vi "Operation Window.vi"(6 "Main UI Message Queue":refnum<queue>, 7 "Pump On?":enum16{"Off", "On", "Not Initialized"}(ring), 8 "error in (no error)":errorcluster, 9 "Graph Notifier":refnum<notifier>, 10 "Message Queues":T24, 11 "Feed Module State Cluster in":T2={"Shared Variables"={"PID 1 Process Variable"="PID1-Mettler Toledo Scale 1", "PID 1 Output"="PID1-Mettler Toledo Scale 1", "PID 1 Setpoint"="PID1-Setpoint", "PID 1 Setpoint SV refnum"="ni.var.psp://localhost/Flow Module 1/PID1-Setpoint", "PID 1 Process Variable SV refnum"="ni.var.psp://localhost/Flow Module 1/PID1-Setpoint", "PID 1 Output SV refnum"="ni.var.psp://localhost/Flow Module 1/PID1-Setpoint"}, "Feed Module Config"={"GUID"="", "Drop Coords"={"Horizontal"=0, "Vertical"=0}, "Process Name"="", "Queue Name"="", "Settings"={"Cycle Period"=500.0, "Ismatech"={"VISA resource name"="", "Simulated?"=TRUE, "Pump Number"=1.0, "Reverse?"=FALSE}, "Masterflex"={"VISA resource name"="", "Simulated?"=TRUE, "Pump Number"=1.0, "Reverse?"=FALSE}, "Mettler"={"VISA resource name"="", "Simulated?"=FALSE}, "Bronkhorst M13 Flow Meter"={"VISA resource name"="", "Simulated?"=TRUE, "Smoothing Steps"=1}, "PID 2 Parameters"={"Input Device"=enum."Default", "Output Device"=enum."Default", "Setpoint"=0.0, "PID gains"={"proportional gain (Kc)"=1.0, "integral time (Ti, min)"=0.01, "derivative time (Td, min)"=0.0}}, "Manual Entry"=0.0, "Auto?"=TRUE, "output range"={"output high"=100.0, "output low"=0.0}, "Tacmina Settings"={"Analog DAQ Task"="", "Digital DAQ Task"=""}, "KNF SIMDOS Settings"={"VISA resource name"="", "Simulated?"=TRUE}, "ASIA Pump C"={"ASIA Pump #"=0, "channel"=0, "Simulated"=FALSE}, "VICI Settings"={"VISA resource name"="", "Simulated?"=TRUE, "Pump Letter"="", "Reverse?"=FALSE}, "FLOM Settings"={"VISA resource name"="", "Simulated?"=TRUE, "Pump Number"=0.0}, "SSI PR/LD Settings"={"VISA resource name"="", "Simulated?"=FALSE}, "Masterflex 75211 Settings"={"Analog DAQ Task"="", "Digital DAQ Task"=""}, "SSI P40 Settings"={"VISA resource name"="", "Simulated?"=TRUE}, "Ismatech 3 Channel Settings"={"VISA resource name"="", "Pump Number"=1, "Channel Number"=0, "Simulated?"=TRUE, "Reverse?"=FALSE}, "Bronkhorst M14 Settings"={"VISA resource name"="", "Simulated?"=FALSE, "Smoothing Steps"=1}}, "Settings Load Count"=0, "OP Load Count"=0}} {"Feed Module Config"."Settings"."Bronkhorst M14 Settings"."Smoothing Steps" min=1 step=1; "Feed Module Config"."Settings"."Ismatech 3 Channel Settings"."Channel Number" min=0 max=3; "Feed Module Config"."Settings"."Ismatech 3 Channel Settings"."Pump Number" min=1; "Feed Module Config"."Settings"."output range"."output low" min=0.0 max=100.0 format="%.2f"; "Feed Module Config"."Settings"."output range"."output high" format="%.2f"; "Feed Module Config"."Settings"."PID 2 Parameters"."PID gains"."derivative time (Td, min)" format="%.3f"; "Feed Module Config"."Settings"."PID 2 Parameters"."PID gains"."integral time (Ti, min)" format="%.3f"; "Feed Module Config"."Settings"."PID 2 Parameters"."PID gains"."proportional gain (Kc)" format="%.3f"; "Feed Module Config"."Settings"."Bronkhorst M13 Flow Meter"."Smoothing Steps" min=1 step=1; "Feed Module Config"."Settings"."ASIA Pump C"."channel" min=0 max=1 step=1; "Feed Module Config"."Settings"."Ismatech"."Pump Number" min=1.0 max=20.0 step=1.0; "Feed Module Config"."Settings"."Masterflex"."Pump Number" min=1.0 max=20.0 step=1.0}) -> (0 "error out":errorcluster, 2 "Need Update":bool, 3 "Feed Module State Cluster out":T2={"Shared Variables"={"PID 1 Process Variable"="PID1-Mettler Toledo Scale 1", "PID 1 Output"="PID1-Mettler Toledo Scale 1", "PID 1 Setpoint"="PID1-Setpoint", "PID 1 Setpoint SV refnum"="ni.var.psp://localhost/Flow Module 1/PID1-Setpoint", "PID 1 Process Variable SV refnum"="ni.var.psp://localhost/Flow Module 1/PID1-Setpoint", "PID 1 Output SV refnum"="ni.var.psp://localhost/Flow Module 1/PID1-Setpoint"}, "Feed Module Config"={"GUID"="", "Drop Coords"={"Horizontal"=0, "Vertical"=0}, "Process Name"="", "Queue Name"="", "Settings"={"Cycle Period"=500.0, "Ismatech"={"VISA resource name"="", "Simulated?"=TRUE, "Pump Number"=1.0, "Reverse?"=FALSE}, "Masterflex"={"VISA resource name"="", "Simulated?"=TRUE, "Pump Number"=1.0, "Reverse?"=FALSE}, "Mettler"={"VISA resource name"="", "Simulated?"=FALSE}, "Bronkhorst M13 Flow Meter"={"VISA resource name"="", "Simulated?"=TRUE, "Smoothing Steps"=1}, "PID 2 Parameters"={"Input Device"=enum."Default", "Output Device"=enum."Default", "Setpoint"=0.0, "PID gains"={"proportional gain (Kc)"=1.0, "integral time (Ti, min)"=0.01, "derivative time (Td, min)"=0.0}}, "Manual Entry"=0.0, "Auto?"=TRUE, "output range"={"output high"=100.0, "output low"=0.0}, "Tacmina Settings"={"Analog DAQ Task"="", "Digital DAQ Task"=""}, "KNF SIMDOS Settings"={"VISA resource name"="", "Simulated?"=TRUE}, "ASIA Pump C"={"ASIA Pump #"=0, "channel"=0, "Simulated"=FALSE}, "VICI Settings"={"VISA resource name"="", "Simulated?"=TRUE, "Pump Letter"="", "Reverse?"=FALSE}, "FLOM Settings"={"VISA resource name"="", "Simulated?"=TRUE, "Pump Number"=0.0}, "SSI PR/LD Settings"={"VISA resource name"="", "Simulated?"=FALSE}, "Masterflex 75211 Settings"={"Analog DAQ Task"="", "Digital DAQ Task"=""}, "SSI P40 Settings"={"VISA resource name"="", "Simulated?"=TRUE}, "Ismatech 3 Channel Settings"={"VISA resource name"="", "Pump Number"=1, "Channel Number"=0, "Simulated?"=TRUE, "Reverse?"=FALSE}, "Bronkhorst M14 Settings"={"VISA resource name"="", "Simulated?"=FALSE, "Smoothing Steps"=1}}, "Settings Load Count"=0, "OP Load Count"=0}} {"Feed Module Config"."Settings"."Bronkhorst M14 Settings"."Smoothing Steps" min=1 step=1; "Feed Module Config"."Settings"."Ismatech 3 Channel Settings"."Channel Number" min=0 max=3; "Feed Module Config"."Settings"."Ismatech 3 Channel Settings"."Pump Number" min=1; "Feed Module Config"."Settings"."output range"."output low" min=0.0 max=100.0 format="%.2f"; "Feed Module Config"."Settings"."output range"."output high" format="%.2f"; "Feed Module Config"."Settings"."PID 2 Parameters"."PID gains"."derivative time (Td, min)" format="%.3f"; "Feed Module Config"."Settings"."PID 2 Parameters"."PID gains"."integral time (Ti, min)" format="%.3f"; "Feed Module Config"."Settings"."PID 2 Parameters"."PID gains"."proportional gain (Kc)" format="%.3f"; "Feed Module Config"."Settings"."Bronkhorst M13 Flow Meter"."Smoothing Steps" min=1 step=1; "Feed Module Config"."Settings"."ASIA Pump C"."channel" min=0 max=1 step=1; "Feed Module Config"."Settings"."Ismatech"."Pump Number" min=1.0 max=20.0 step=1.0; "Feed Module Config"."Settings"."Masterflex"."Pump Number" min=1.0 max=20.0 step=1.0})   [LabVIEW 2018, in "Feed Module.lvlib"]
uses:
  Feed Module/Feed Module.lvlib
  Feed Module/Controls/Feed Message Queues.ctl
  support/Message Queue/Message Cluster.ctl
  Feed Module/Controls/Feed Module State Cluster.ctl
  Feed Module/Controls/Feed Module Shared Variable Cluster.ctl
  Feed Module/Controls/Feed Module Config Cluster.ctl
  <vilib>/Utility/miscctls.llb/LVPoint32TypeDef.ctl
  Feed Module/Controls/Feed Module Settings Cluster.ctl
  Ismatec ISM 831C/Controls/Ismatech ISM831C Settings Cluster.ctl
  Masterflex 7550-30/Controls/Settings Cluster.ctl
  Mettler Toledo/Controls/Settings Cluster.ctl
  Bronkhorst M13 Flow Meter/Settings Cluster.ctl
  Measure Instrument/PID 2 Parameters Cluster.ctl
  Measure Instrument/PID Input Enum.ctl
  Measure Instrument/PID 2 Output Enum.ctl
  Tacmina QI/Tacmina QI DAQ Setting.ctl
  KNF Pump/Settings Cluster plus SIMDOS.ctl
  ASIA Pump/Pump Settings.ctl
  VICI M50 Party Mode/Settings Cluster.ctl
  FLOM Pump/Settings Cluster.ctl
  SSI PR Class/SSI PR or LD Settings Cluster.ctl
  Masterflex 75211/Masterflex 75211 DAQ Setting.ctl
  SSI PR Class/SSI P40 Settings Cluster.ctl
  Ismatec 78001/Ismatec 4083.ctl
  Bronkhorst M14 Flow Meter/Settings Cluster.ctl
  Config Module/Controls/OP Window Display.ctl
  support/Message Queue/Enqueue Message (Single).vi
  support/Message Queue/Message Queue.lvlib
  support/Support Library.lvlib
  Settings/Settings Dialog.vi
  Settings/Settings.lvlib
  Ismatec ISM 831C/Ismatec ISM 831C.lvlib
  Masterflex 7550-30/Masterflex 7550-30.lvlib
  Mettler Toledo/Mettler Toledo.lvlib
  Bronkhorst M13 Flow Meter/Bronkhorst M13 Flow Meter.lvlib
  Tacmina QI/Tacmina QI.lvlib
  KNF Pump/KNF SIMDOS.lvlib
  ASIA Pump.lvlib
  VICI M50 Party Mode/VICI M6 M50 Party Mode.lvlib
  FLOM Pump/FLOM Pump.lvlib
  SSI PR Class/SSI PR or LD Pump.lvlib
  Masterflex 75211/Masterflex 75211.lvlib
  SSI PR Class/SSI P40 Pump.lvlib
  Ismatec 78001/Ismatec 4308.lvlib
  Bronkhorst M14 Flow Meter/Bronkhorst M14 Flow Meter.lvlib
panel:
  out "Smoothed Array":dbl[](array[numeric])
  out "Start button status":T1(ring)
  out "Started":bool
  out "Updated":bool
  out "Flow":dbl caption="gm/min" format="%.2f"
  out "Data":waveform(dbl)[](graph)
  in  "Auto?":bool=TRUE
  in  "Manual Entry":dbl step=0.1 format="%#_6f"
  in  "Setpoint":dbl
  in  "Cancel Button":bool
  in  "OK Button":bool
  in  "Start":bool
  in  "Settings":bool
  in  "Stop":bool
  # "Output Instruments"
  # "Input Instruments"
  # "Output Instruments"
  # "Input Instruments"
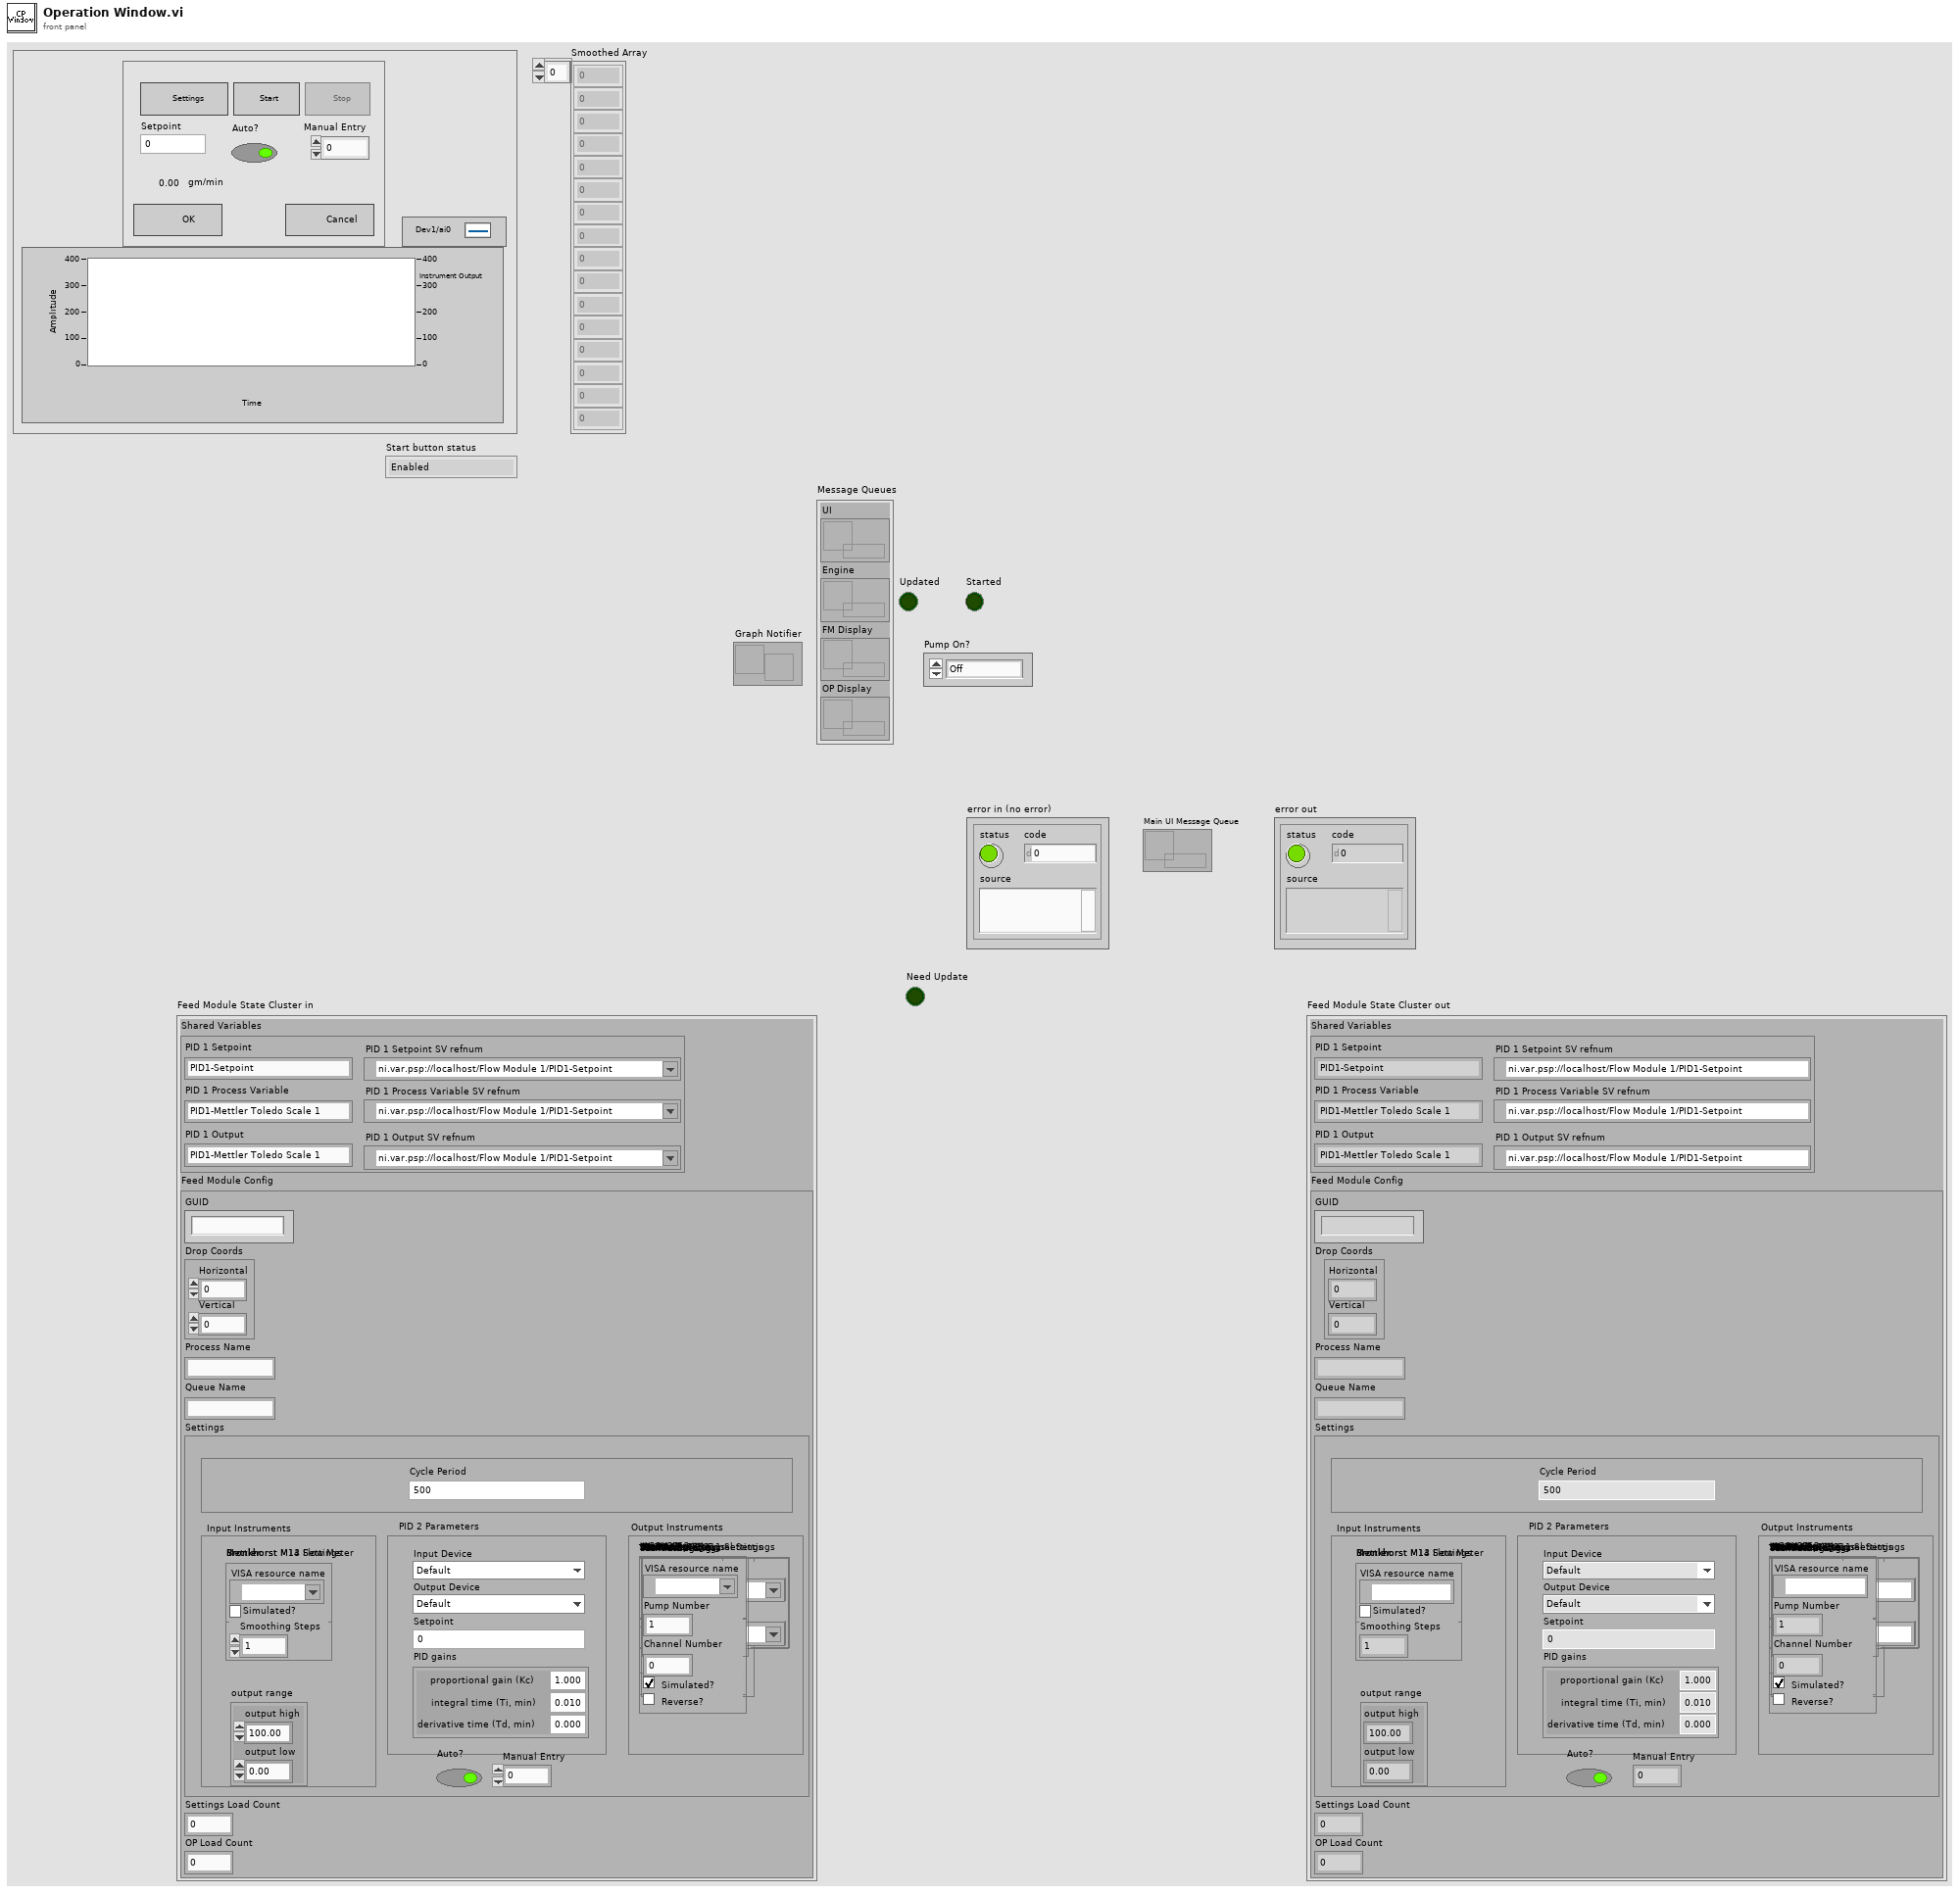
[diagram p1: front panel]
types:
  T1 = enum8{"Enabled", "Disabled", "Disabled and Grayed Out"}
  T2 = typedef "Feed Module.lvlib/Feed Module State Cluster.ctl" = cluster{"Shared Variables":T3, "Feed Module Config":T4}
  T3 = typedef "Feed Module.lvlib/Feed Module Shared Variable Cluster.ctl" = cluster{"PID 1 Process Variable":string, "PID 1 Output":string, "PID 1 Setpoint":string, "PID 1 Setpoint SV refnum":refnum<k21>, "PID 1 Process Variable SV refnum":refnum<k21>, "PID 1 Output SV refnum":refnum<k21>}
  T4 = typedef "Feed Module.lvlib/Feed Module Config Cluster.ctl" = cluster{"GUID":string, "Drop Coords":T5, "Process Name":string, "Queue Name":string, "Settings":T6, "Settings Load Count":i32, "OP Load Count":i32}
  T5 = typedef "LVPoint32TypeDef.ctl" = cluster{"Horizontal":i32, "Vertical":i32}
  T6 = typedef "Feed Module.lvlib/Feed Module Settings Cluster.ctl" = cluster{"Cycle Period":dbl, "Ismatech":T7, "Masterflex":T8, "Mettler":T9, "Bronkhorst M13 Flow Meter":T10, "PID 2 Parameters":T11, "Manual Entry":dbl, "Auto?":bool, "output range":cluster{"output high":dbl, "output low":dbl}, "Tacmina Settings":T14, "KNF SIMDOS Settings":T15, "ASIA Pump C":T16, "VICI Settings":T17, "FLOM Settings":T18, "SSI PR/LD Settings":T19, "Masterflex 75211 Settings":T20, "SSI P40 Settings":T21, "Ismatech 3 Channel Settings":T22, "Bronkhorst M14 Settings":T23}
  T7 = typedef "Ismatec ISM 831C.lvlib/Ismatech ISM831C Settings Cluster.ctl" = cluster{"VISA resource name":refnum<visa-resource-name>, "Simulated?":bool, "Pump Number":dbl, "Reverse?":bool}
  T8 = typedef "Masterflex 7550-30.lvlib/Settings Cluster.ctl" = cluster{"VISA resource name":refnum<visa-resource-name>, "Simulated?":bool, "Pump Number":dbl, "Reverse?":bool}
  T9 = typedef "Mettler Toledo.lvlib/Settings Cluster.ctl" = cluster{"VISA resource name":refnum<visa-resource-name>, "Simulated?":bool}
  T10 = typedef "Bronkhorst M13 Flow Meter.lvlib/Settings Cluster.ctl" = cluster{"VISA resource name":refnum<visa-resource-name>, "Simulated?":bool, "Smoothing Steps":i32}
  T11 = typedef "PID 2 Parameters Cluster.ctl" = cluster{"Input Device":T12, "Output Device":T13, "Setpoint":dbl, "PID gains":cluster{"proportional gain (Kc)":dbl, "integral time (Ti, min)":dbl, "derivative time (Td, min)":dbl}}
  T12 = typedef "PID Input Enum.ctl" = enum16{"Default", "Bronkhorst M13", "Bronkhorst M14", "Scale Rate of Change"}
  T13 = typedef "PID 2 Output Enum.ctl" = enum16{"Default", "Ismatec ISM 4308", "Ismatec ISM 831C", "Masterflex 7550-30", "VICI", "Tacmina QI", "KNF SIMDOS", "ASIA Type C", "FLOM UI-22-11", "SSI PR/LD", "SSI P40", "Masterflex 75211-70"}
  T14 = typedef "Tacmina QI.lvlib/Tacmina QI DAQ Setting.ctl" = cluster{"Analog DAQ Task":refnum<k21>, "Digital DAQ Task":refnum<k21>}
  T15 = typedef "KNF SIMDOS.lvlib/Settings Cluster plus SIMDOS.ctl" = cluster{"VISA resource name":refnum<visa-resource-name>, "Simulated?":bool}
  T16 = typedef "ASIA Pump.lvlib/Pump Settings.ctl" = cluster{"ASIA Pump #":i32, "channel":i32, "Simulated":bool}
  T17 = typedef "VICI M6 M50 Party Mode.lvlib/Settings Cluster.ctl" = cluster{"VISA resource name":refnum<visa-resource-name>, "Simulated?":bool, "Pump Letter":string, "Reverse?":bool}
  T18 = typedef "FLOM Pump.lvlib/Settings Cluster.ctl" = cluster{"VISA resource name":refnum<visa-resource-name>, "Simulated?":bool, "Pump Number":dbl}
  T19 = typedef "SSI PR or LD Pump.lvlib/SSI PR or LD Settings Cluster.ctl" = cluster{"VISA resource name":refnum<visa-resource-name>, "Simulated?":bool}
  T20 = typedef "Masterflex 75211.lvlib/Masterflex 75211 DAQ Setting.ctl" = cluster{"Analog DAQ Task":refnum<k21>, "Digital DAQ Task":refnum<k21>}
  T21 = typedef "SSI P40 Pump.lvlib/SSI P40 Settings Cluster.ctl" = cluster{"VISA resource name":refnum<visa-resource-name>, "Simulated?":bool}
  T22 = typedef "Ismatec 4308.lvlib/Ismatec 4083.ctl" = cluster{"VISA resource name":refnum<visa-resource-name>, "Pump Number":i16, "Channel Number":i16, "Simulated?":bool, "Reverse?":bool}
  T23 = typedef "Bronkhorst M14 Flow Meter.lvlib/Settings Cluster.ctl" = cluster{"VISA resource name":refnum<visa-resource-name>, "Simulated?":bool, "Smoothing Steps":i32}
  T24 = typedef "Feed Module.lvlib/Feed Message Queues.ctl" = cluster{"UI":refnum<queue>, "Engine":refnum<queue>, "FM Display":refnum<queue>, "OP Display":refnum<queue>}
  T25 = typedef "Feed Module.lvlib/OP Window Display.ctl" = cluster{"Flow":dbl, "Manual":dbl, "Pump Status":u16, "Smoothed Array":dbl[]}
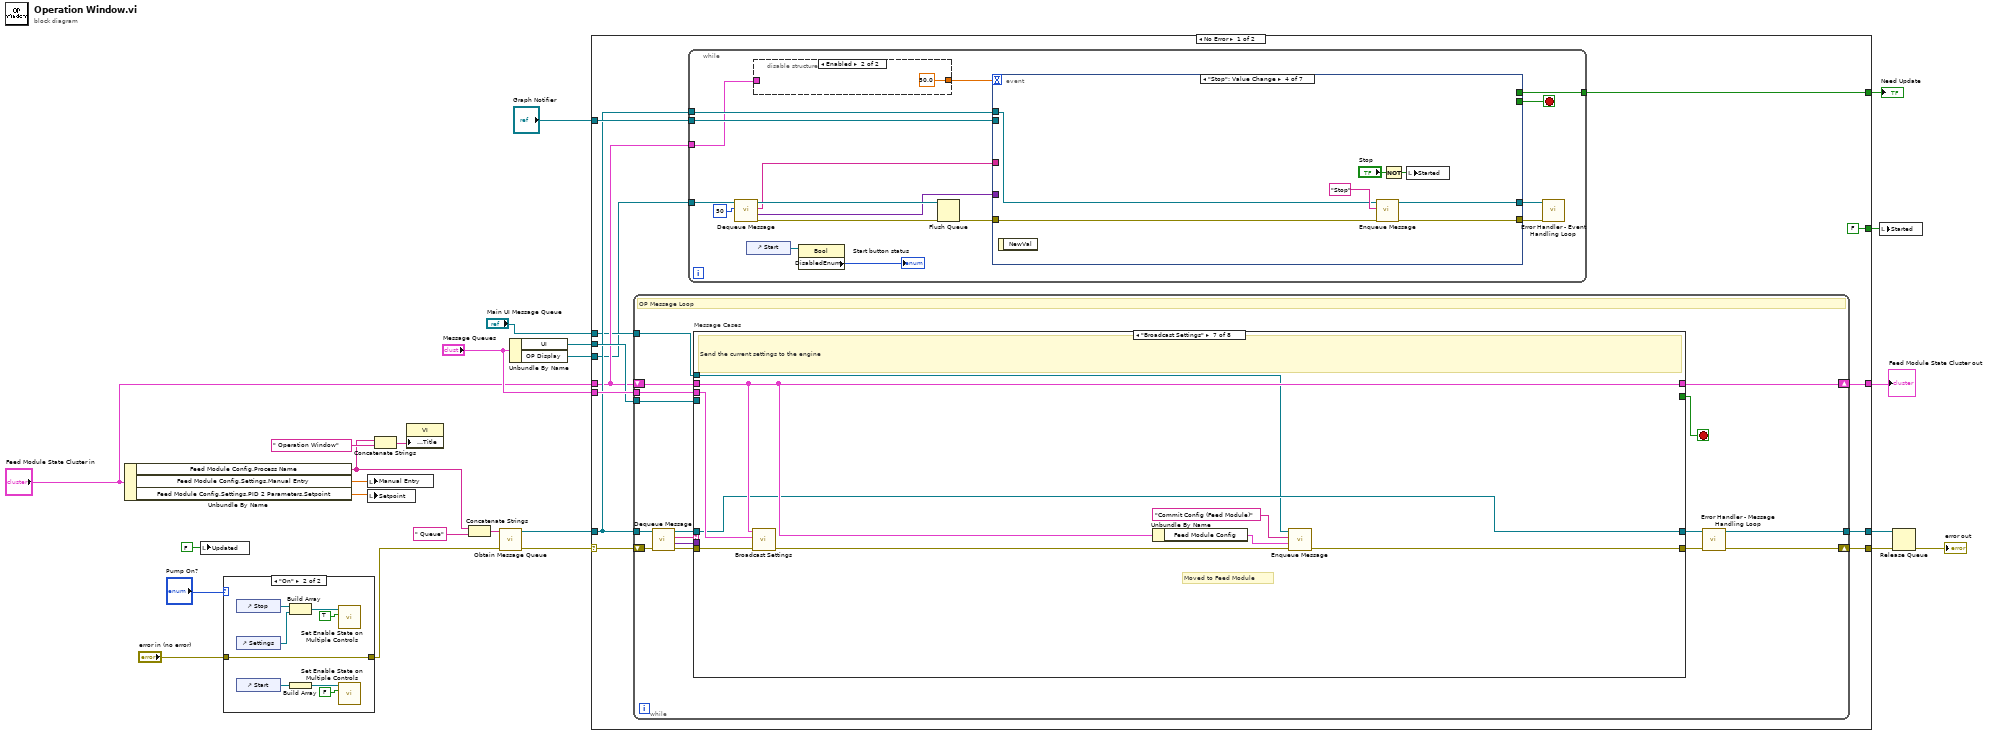
[diagram p0: block diagram]
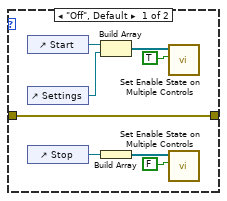
[diagram p2: hidden frame]
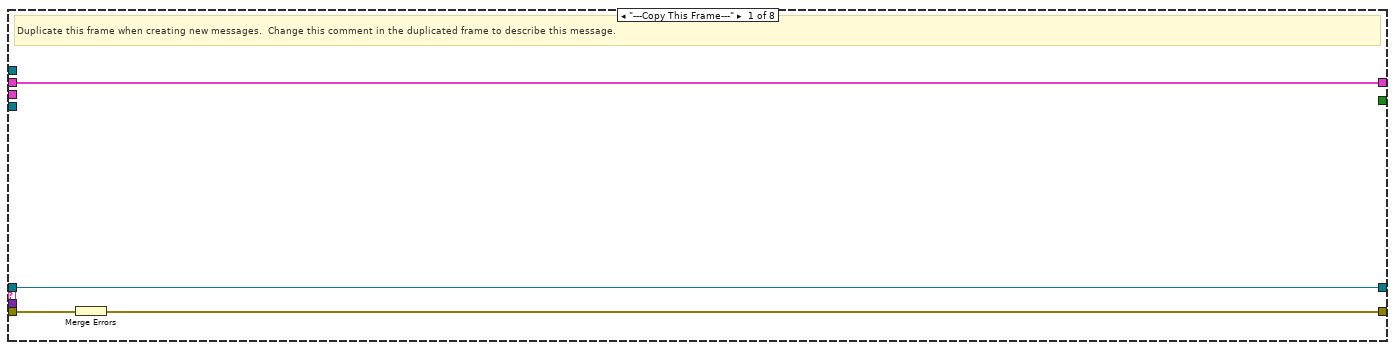
[diagram p3: hidden frame]
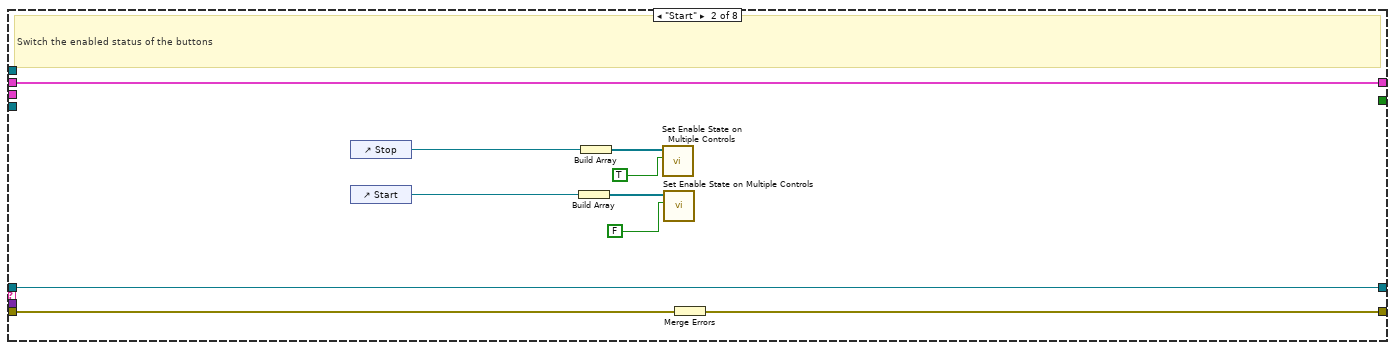
[diagram p4: hidden frame]
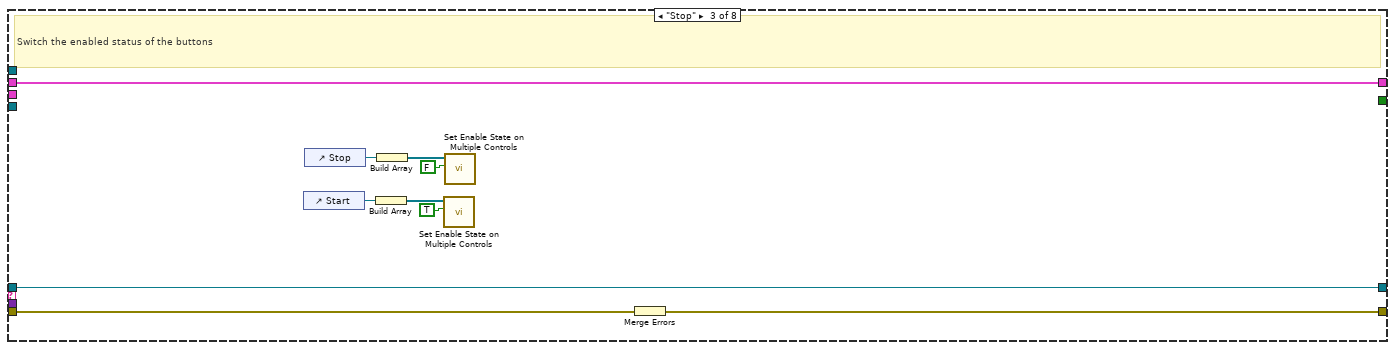
[diagram p5: hidden frame]
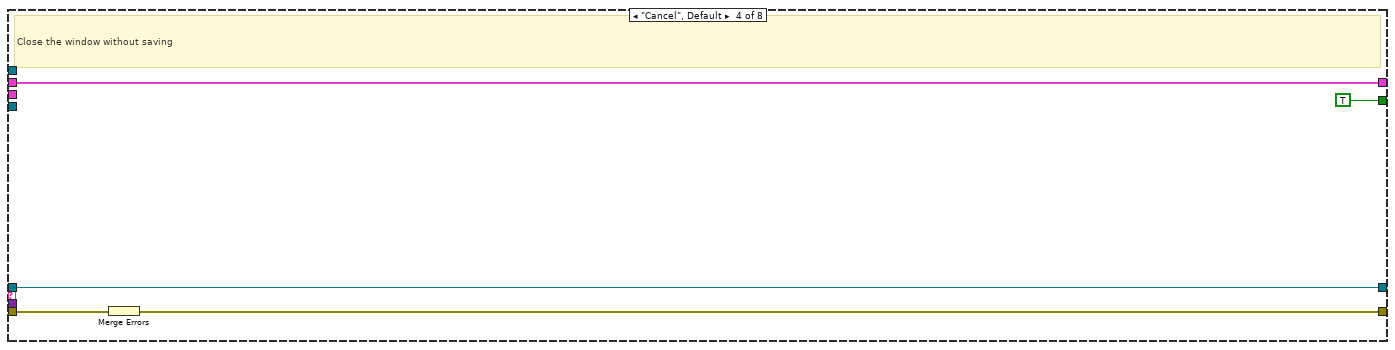
[diagram p6: hidden frame]
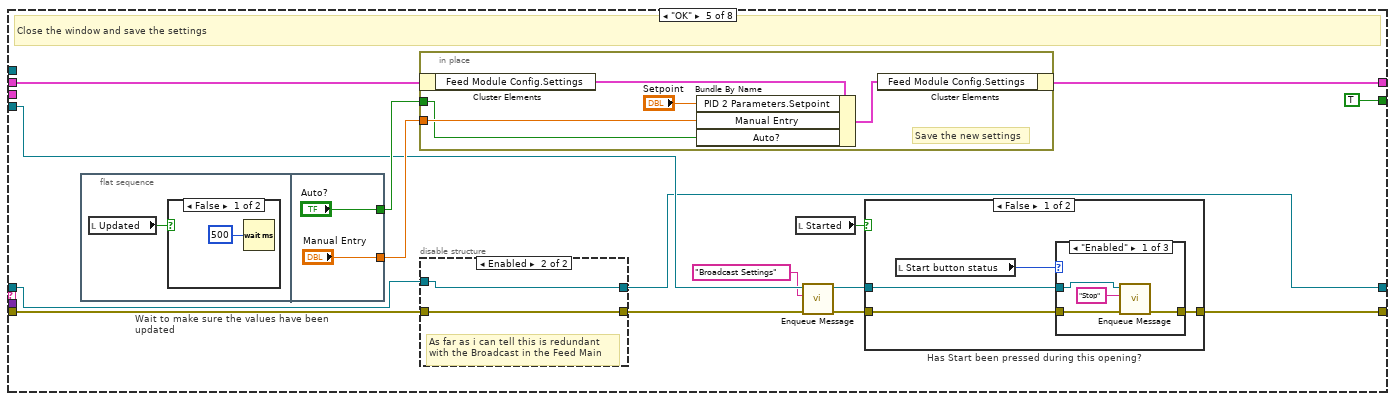
[diagram p7: hidden frame]
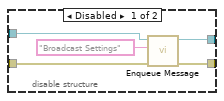
[diagram p8: hidden frame]
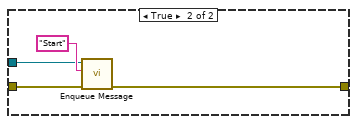
[diagram p11: hidden frame]
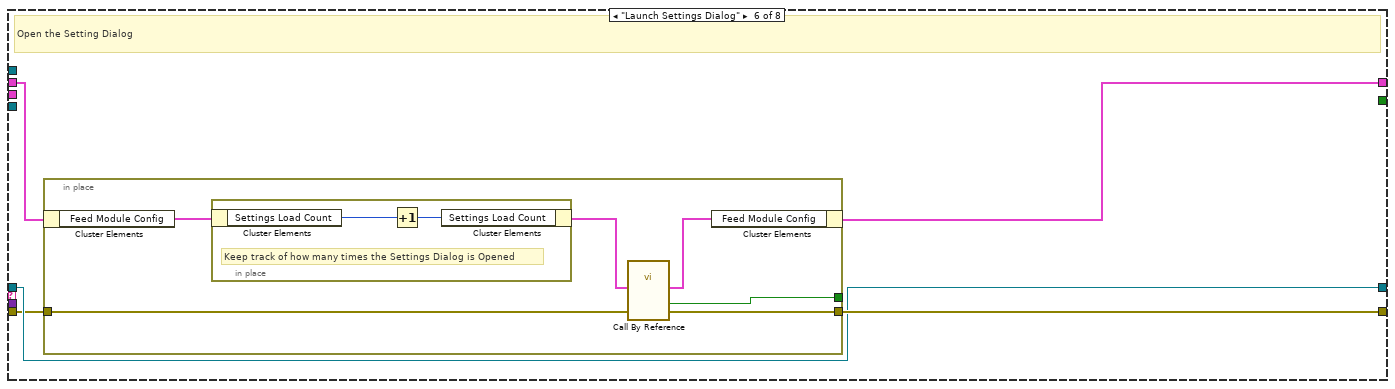
[diagram p13: hidden frame]
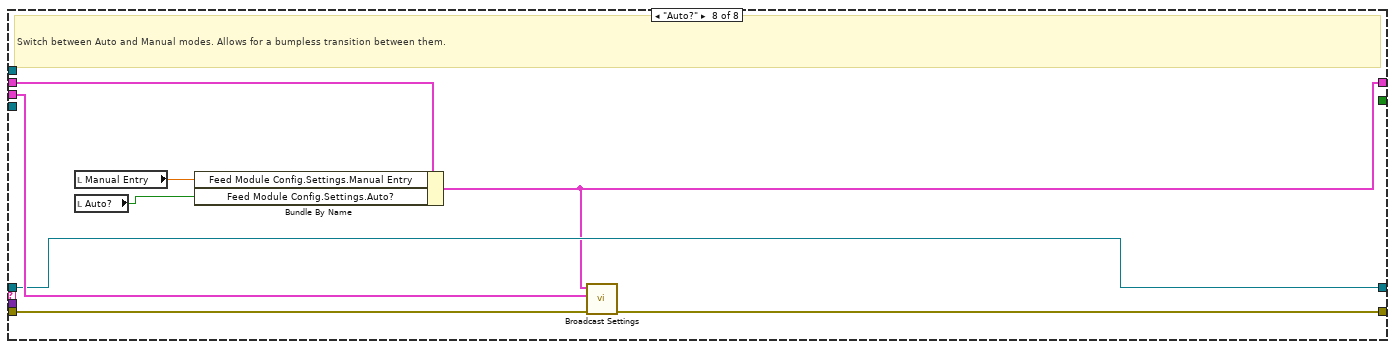
[diagram p14: hidden frame]
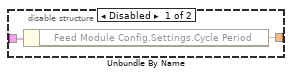
[diagram p15: hidden frame]
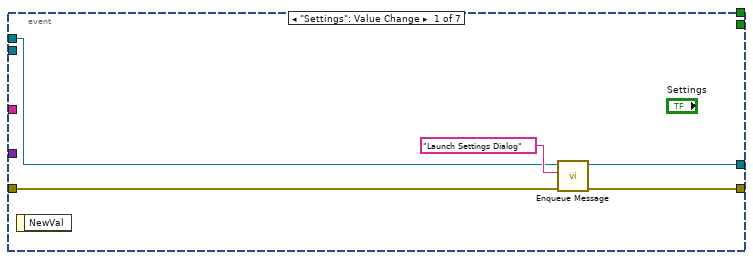
[diagram p16: hidden frame]
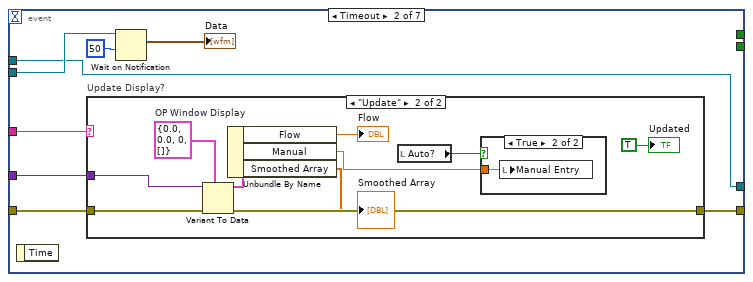
[diagram p17: hidden frame]
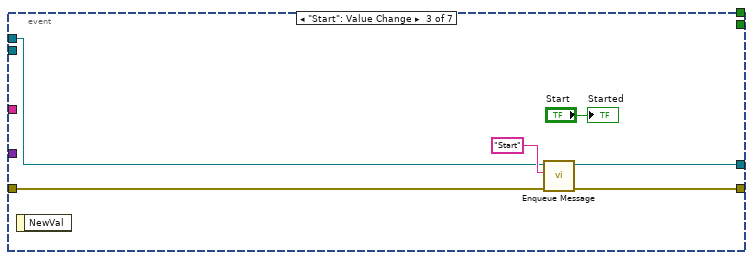
[diagram p20: hidden frame]
diagram:
  n1 = Unbundle By Name("Feed Module State Cluster in") -> ("Feed Module Config.Process Name"=w11:string, "Feed Module Config.Settings.Manual Entry"=w17:dbl, "Feed Module Config.Settings.PID 2 Parameters.Setpoint"=w15:dbl)
  n2 = local write "Updated"(FALSE ("Boolean")) -> ()
  n3 = case shown="\"On\"" "Pump On?" {
    tunnel: "error in (no error)" -> [w26 w34]
    tunnel: [w26 w34] -> w2
    frame "Off", Default {
      n4 = control-ref of="Start"() -> (w29:refnum<vi>)
      n5 = control-ref of="Settings"() -> (w28:refnum<vi>)
      n6 = control-ref of="Stop"() -> (w27:refnum<vi>)
      n7 = Build Array(w29, w28) -> (w32:refnum<vi>[])
      n8 = Build Array(w27) -> (w31:refnum<vi>[])
      n9 = call "Set Enable State on Multiple Controls.vi"("Enable?"=TRUE, "Controls"=w32) -> ()  [unwired: 10 in]
      n10 = call "Set Enable State on Multiple Controls.vi"("Enable?"=FALSE, "Controls"=w31) -> ()  [unwired: 10 in]
    }
    frame "On" {
      n11 = control-ref of="Stop"() -> (w36:refnum<vi>)
      n12 = control-ref of="Settings"() -> (w35:refnum<vi>)
      n13 = control-ref of="Start"() -> (w37:refnum<vi>)
      n14 = Build Array(w36, w35) -> (w39:refnum<vi>[])
      n15 = Build Array(w37) -> (w40:refnum<vi>[])
      n16 = call "Set Enable State on Multiple Controls.vi"("Enable?"=TRUE, "Controls"=w39) -> ()  [unwired: 10 in]
      n17 = call "Set Enable State on Multiple Controls.vi"("Enable?"=FALSE, "Controls"=w40) -> ()  [unwired: 10 in]
    }
  }
  n18 = local write "Manual Entry"(w17) -> ()
  n19 = local write "Setpoint"(w15) -> ()
  n20 = Concatenate Strings(w11, " Operation Window" ("string")) -> (w10:string)
  n21 = property class="VI"("Front Panel.Title"=w10) -> ()  [unwired: 2 in, 2 out]
  n22 = Concatenate Strings(w11, " Queue" ("string")) -> (w14:string)
  n23 = call "Obtain Message Queue.vi"("error in (no error)"=w2, "name (unnamed)"=w14) -> ("error out"=w7:errorcluster, "Message Queue"=w23:refnum<queue>)  [unwired: 8 in]
  n24 = Unbundle By Name("Message Queues") -> ("UI"=w21:refnum<queue>, "OP Display"=w18:refnum<queue>)
  n25 = case shown="No Error" w7 {
    selector: w7 -> [w43 w256]
    tunnel: [w47 w256] -> w5
    tunnel: [w54 FALSE] -> w25
    tunnel: w23 -> [w49 w252]
    tunnel: "Feed Module State Cluster in" -> [w48 w254]
    tunnel: [w53 w254] -> w19
    tunnel: "Message Queues" -> [w52 _]
    tunnel: "Graph Notifier" -> [w51 _]
    tunnel: w21 -> [w50 _]
    tunnel: "Main UI Message Queue" -> [w46 _]
    tunnel: w18 -> [w45 _]
    tunnel: [FALSE FALSE] -> w8
    tunnel: [w42 w252] -> w6
    frame No Error {
      n26 = while {
        shift-right: [w59] -> w47
        shift-left: w43 -> [w62]
        tunnel: w49 -> [w61]
        tunnel: w52 -> [w63]
        shift-right: [w64] -> w53
        shift-left: w48 -> [w60]
        tunnel: w50 -> [w58]
        tunnel: w46 -> [w56]
        tunnel: [w55] -> w42
        stop <- w65 stop-if-true
        # "OP Message Loop"
        n27 = call "Dequeue Message.vi"("error in (no error)"=w62, "Message Queue"=w61) -> ("error out"=w66:errorcluster, "Message Data"=w69:variant, "Message"=w70:string, "dup Message Queue"=w67:refnum<queue>)  [unwired: 6 in]
        n28 = case "Message Cases" shown="\"Broadcast Settings\"" w70 {
          tunnel: w67 -> [w71 w75 w85 w95 w103 w148 w163 w172]
          tunnel: w66 -> [w74 w84 w94 w99 w102 w147 w165 w173]
          tunnel: [w73 w83 w93 w98 w109 w149 w162 w167] -> w68
          tunnel: w69 -> [_ _ _ _ _ _ _ _]
          tunnel: [_ _ _ TRUE TRUE _ _ _] -> w65
          tunnel: w60 -> [w72 w76 w92 w96 w105 w146 w164 w169]
          tunnel: [w72 w76 w92 w96 w104 w145 w164 w168] -> w64
          tunnel: w63 -> [_ _ _ _ _ _ w166 w174]
          tunnel: w58 -> [_ _ _ _ w111 _ _ _]
          tunnel: [w71 w75 w85 w95 w101 w148 w163 w172] -> w57
          tunnel: w56 -> [_ _ _ _ _ _ w160 _]
          frame "---Copy This Frame---" {
            # "Duplicate this frame when creating new messages.  Change this comment in the duplicated frame to describe this message."
            n29 = Merge Errors(w74) -> (w73:errorcluster)
          }
          frame "Start" {
            # "Switch the enabled status of the buttons"
            n30 = control-ref of="Stop"() -> (w81:refnum<vi>)
            n31 = control-ref of="Start"() -> (w82:refnum<vi>)
            n32 = Build Array(w82) -> (w79:refnum<vi>[])
            n33 = Build Array(w81) -> (w80:refnum<vi>[])
            n34 = call "Set Enable State on Multiple Controls.vi"("Enable?"=TRUE, "Controls"=w80) -> ()  [unwired: 10 in]
            n35 = call "Set Enable State on Multiple Controls.vi"("Enable?"=FALSE, "Controls"=w79) -> ()  [unwired: 10 in]
            n36 = Merge Errors(w84) -> (w83:errorcluster)
          }
          frame "Stop" {
            # "Switch the enabled status of the buttons"
            n37 = control-ref of="Start"() -> (w91:refnum<vi>)
            n38 = control-ref of="Stop"() -> (w88:refnum<vi>)
            n39 = Build Array(w91) -> (w90:refnum<vi>[])
            n40 = Build Array(w88) -> (w87:refnum<vi>[])
            n41 = call "Set Enable State on Multiple Controls.vi"("Enable?"=TRUE, "Controls"=w90) -> ()  [unwired: 10 in]
            n42 = call "Set Enable State on Multiple Controls.vi"("Enable?"=FALSE, "Controls"=w87) -> ()  [unwired: 10 in]
            n43 = Merge Errors(w94) -> (w93:errorcluster)
          }
          frame "Cancel", Default {
            # "Close the window without saving"
            n44 = Merge Errors(w99) -> (w98:errorcluster)
          }
          frame "OK" {
            # "Close the window and save the settings"
            n45 = flat-sequence "Wait to make sure the values have been updated" {
              tunnel: ["Manual Entry"] -> w113
              tunnel: ["Auto?"] -> w112
              frame #0 {
                n46 = local read "Updated"() -> (w141:bool)
                n47 = case shown="False" w141 {
                  frame False {
                    n48 = Wait (ms)(milliseconds to wait=u32 500) -> ()  [unwired: 1 out]
                  }
                  frame True {
                  }
                }
              }
              frame #1 {
              }
            }
            n49 = in-place {
              in-place-border: w113 -> [w125]
              in-place-border: w112 -> [w124]
              # "Save the new settings"
              n50 = in-place-cluster #1(w105) -> ("Feed Module Config.Settings"=w123:T6)
              n51 = Bundle By Name(cluster=w123, "PID 2 Parameters.Setpoint"="Setpoint", "Manual Entry"=w125, "Auto?"=w124) -> (w122:T6)
              n52 = in-place-cluster #1("Feed Module Config.Settings"=w122) -> (w104:T2)
            }
            n53 = disable-structure shown="Enabled" {
              disable-tunnel: w103 -> [w119 w121]
              disable-tunnel: w102 -> [w118 w120]
              disable-tunnel: [w117 w121] -> w101
              disable-tunnel: [w116 w120] -> w100
              frame Disabled {
                n54 = call-poly "Enqueue Message.vi"("error in (no error)"=w118, "Message"="Broadcast Settings", "Message Queue"=w119) -> ("error out"=w116:errorcluster, "dup Message Queue"=w117:refnum<queue>)  [unwired: 7 in]
              }
              frame Enabled {
                # "As far as i can tell this is redundant\nwith the Broadcast in the Feed Main"
              }
            }
            n55 = local read "Started"() -> (w110:bool)
            n56 = call-poly "Enqueue Message.vi"("error in (no error)"=w100, "Message"="Broadcast Settings", "Message Queue"=w111) -> ("error out"=w106:errorcluster, "dup Message Queue"=w107:refnum<queue>)  [unwired: 7 in]
            n57 = case "Has Start been pressed during this opening?" shown="False" w110 {
              tunnel: w107 -> [w128 w139]
              tunnel: w106 -> [w129 w138]
              tunnel: [w130 w137] -> w109
              frame False {
                n58 = local read "Start button status"() -> (w127:T1)
                n59 = case shown="\"Enabled\"" w127 {
                  tunnel: [w133 w135 w136] -> w130
                  tunnel: w129 -> [w132 w135 w136]
                  tunnel: w128 -> [w131 _ _]
                  frame "Enabled" {
                    n60 = call-poly "Enqueue Message.vi"("error in (no error)"=w132, "Message"="Stop", "Message Queue"=w131) -> ("error out"=w133:errorcluster)  [unwired: 7 in, 1 out]
                  }
                  frame "Disabled" {
                  }
                  frame "Disabled and Grayed Out" {
                  }
                }
              }
              frame True {
                n61 = call-poly "Enqueue Message.vi"("error in (no error)"=w138, "Message"="Start", "Message Queue"=w139) -> ("error out"=w137:errorcluster)  [unwired: 7 in, 1 out]
              }
            }
          }
          frame "Launch Settings Dialog" {
            # "Open the Setting Dialog"
            n62 = in-place {
              in-place-border: [w155] -> _
              in-place-border: [w154] -> w149
              in-place-border: w147 -> [w153]
              n63 = in-place-cluster #2(w146) -> ("Feed Module Config"=w150:T4)
              n64 = in-place {
                # "Keep track of how many times the Settings Dialog is Opened"
                n65 = in-place-cluster #3(w150) -> ("Settings Load Count"=w157:i32)
                n66 = Increment(x=w157) -> (x+1=w156:i32)
                n67 = in-place-cluster #3("Settings Load Count"=w156) -> (w152:T4)
              }
              n68 = call-by-ref "?"("error in (no error)"=w153, "Feed Module Config in"=w152) -> ("error out"=w154:errorcluster, "Cancelled?"=w155:bool, "Feed Module Config out"=w151:T4)  [unwired: 8 in, 3 out]
              n69 = in-place-cluster #2("Feed Module Config"=w151) -> (w145:T2)
            }
          }
          frame "Broadcast Settings" {
            # "Moved to Feed Module"
            # "Send the current settings to the engine"
            n70 = call "Broadcast Settings.vi"("error in (no error)"=w165, "Message Queues"=w166, "Feed Module State Cluster in"=w164) -> ("error out"=w161:errorcluster)  [unwired: 8 in]
            n71 = Unbundle By Name(w164) -> ("Feed Module Config"=w159:T4)
            n72 = call-poly "Enqueue Message.vi"("error in (no error)"=w161, "Message Data"=w159, "Message"="Commit Config (Feed Module)", "Message Queue"=w160) -> ("error out"=w162:errorcluster)  [unwired: 6 in, 1 out]
          }
          frame "Auto?" {
            # "Switch between Auto and Manual modes. Allows for a bumpless transition between them."
            n73 = local read "Manual Entry"() -> (w171:dbl)
            n74 = local read "Auto?"() -> (w170:bool)
            n75 = Bundle By Name(cluster=w169, "Feed Module Config.Settings.Manual Entry"=w171, "Feed Module Config.Settings.Auto?"=w170) -> (w168:T2)
            n76 = call "Broadcast Settings.vi"("error in (no error)"=w173, "Message Queues"=w174, "Feed Module State Cluster in"=w168) -> ("error out"=w167:errorcluster)  [unwired: 8 in]
          }
        }
        n77 = call "Error Handler - Message Handling Loop.vi"("error in (no error)"=w68, "Message Queue"=w57) -> ("dup error in"=w59:errorcluster, "dup Message Queue"=w55:refnum<queue>)  [unwired: 8 in]
      }
      n78 = while {
        tunnel: [w188] -> w54
        tunnel: w49 -> [w187]
        tunnel: w51 -> [w186]
        tunnel: w48 -> [w184]
        tunnel: w45 -> [w183]
        stop <- w189 stop-if-true
        n79 = call "Dequeue Message.vi"("timeout in ms (-1)"=50, "Message Queue"=w183) -> ("error out"=w181:errorcluster, "Message Data"=w178:variant, "Message"=w179:string, "dup Message Queue"=w180:refnum<queue>)  [unwired: 6 in]
        n80 = control-ref of="Start"() -> (w176:refnum<vi>)
        n81 = disable-structure shown="Enabled" {
          disable-tunnel: [w193 50.0 ("Cycle Period")] -> w185
          disable-tunnel: w184 -> [w192 _]
          frame Disabled {
            n82 = Unbundle By Name(w192) -> ("Feed Module Config.Settings.Cycle Period"=w193:dbl)
          }
          frame Enabled {
          }
        }
        n83 = property class="Bool"(reference=w176) -> ("DisabledEnum"=→"Start button status":T1)  [unwired: 1 in, 2 out]
        n84 = Flush Queue(queue=w180, error in (no error)=w181) -> (error out=w177:errorcluster)  [unwired: 2 out]
        n85 = event shown="[3] \"Stop\": Value Change" {
          selector: _ -> [_ _ _ _ _ _ _]
          dyn-events: _ -> [_ _ _ _ _ _ _]
          timeout: w185 -> [_ _ _ _ _ _ _]
          tunnel: [w198 w200 w222 w230 w235 w242 w250] -> w191
          tunnel: [w197 w201 w223 w229 w234 w241 w249] -> w190
          tunnel: [_ _ _ _ _ TRUE ("Priority Message? (F)") w248] -> w189
          tunnel: [_ _ _ _ _ FALSE ("Priority Message? (F)") w248] -> w188
          tunnel: w187 -> [w196 w200 w224 w231 w236 w239 w247]
          tunnel: w186 -> [_ w206 _ _ _ _ _]
          tunnel: w179 -> [_ w204 _ _ _ _ _]
          tunnel: w178 -> [_ w203 _ _ _ _ _]
          tunnel: w177 -> [w195 w202 w220 w226 w233 w238 w246]
          event "Settings": Value Change {
            n86 = event-data() -> ()  [unwired: 1 in, 1 out]
            n87 = call-poly "Enqueue Message.vi"("error in (no error)"=w195, "Message"="Launch Settings Dialog", "Message Queue"=w196) -> ("error out"=w197:errorcluster, "dup Message Queue"=w198:refnum<queue>)  [unwired: 7 in]
          }
          event Timeout {
            n88 = event-data() -> ()  [unwired: 1 in, 1 out]
            n89 = case "Update Display?" shown="\"Update\"" w204 {
              tunnel: w203 -> [_ w218]
              tunnel: w202 -> [w208 w211]
              tunnel: [w208 w210] -> w201
              frame "False", Default {
              }
              frame "Update" {
                w217 = T25 {"Flow"=0.0, "Manual"=0.0, "Pump Status"=0, "Smoothed Array"=[]}  # OP Window Display
                n90 = Variant To Data(error in=w211, type=w217, Variant=w218) -> (data=w216:T25, error out=w210:errorcluster)
                n91 = Unbundle By Name(w216) -> ("Flow"=→"Flow":dbl, "Manual"=w214:dbl, "Smoothed Array"=→"Smoothed Array":dbl[])
                n92 = local read "Auto?"() -> (w213:bool)
                n93 = case shown="True" w213 {
                  tunnel: w214 -> [_ w219]
                  frame False {
                  }
                  frame True {
                    n94 = local write "Manual Entry"(w219) -> ()
                  }
                }
                "Updated" <- TRUE ("Boolean")
              }
            }
            n95 = Wait on Notification(notifier=w206, timeout in ms (-1)=50) -> (notification=→"Data":waveform(dbl)[])  [unwired: 2 in, 3 out]
          }
          event "Start": Value Change {
            n96 = event-data() -> ()  [unwired: 1 in, 1 out]
            n97 = call-poly "Enqueue Message.vi"("error in (no error)"=w220, "Message"="Start", "Message Queue"=w224) -> ("error out"=w223:errorcluster, "dup Message Queue"=w222:refnum<queue>)  [unwired: 7 in]
            "Started" <- "Start"
          }
          event "Stop": Value Change {
            n98 = event-data() -> ()  [unwired: 1 in, 1 out]
            n99 = call-poly "Enqueue Message.vi"("error in (no error)"=w226, "Message"="Stop", "Message Queue"=w231) -> ("error out"=w229:errorcluster, "dup Message Queue"=w230:refnum<queue>)  [unwired: 7 in]
            n100 = Not(x="Stop") -> (.not. x?=w227:bool)
            n101 = local write "Started"(w227) -> ()
          }
          event "Auto?": Value Change {
            n102 = event-data() -> ()  [unwired: 1 in, 1 out]
            n103 = call-poly "Enqueue Message.vi"("error in (no error)"=w233, "Message"="Auto?", "Message Queue"=w236) -> ("error out"=w234:errorcluster, "dup Message Queue"=w235:refnum<queue>)  [unwired: 7 in]
          }
          event "Cancel Button": Value Change {
            n104 = event-data() -> ()  [unwired: 1 in, 1 out]
            n105 = call-poly "Enqueue Message.vi"("Priority Message? (F)"=TRUE, "error in (no error)"=w238, "Message"="Cancel", "Message Queue"=w239) -> ("error out"=w241:errorcluster, "dup Message Queue"=w242:refnum<queue>)  [unwired: 6 in]
          }
          event "OK Button": Value Change {
            w248 = TRUE
            n106 = event-data() -> ()  [unwired: 1 in, 1 out]
            n107 = call-poly "Enqueue Message.vi"("error in (no error)"=w246, "Message"="OK", "Message Queue"=w247) -> ("error out"=w249:errorcluster, "dup Message Queue"=w250:refnum<queue>)  [unwired: 7 in]
          }
        }
        n108 = call "Error Handler - Event Handling Loop.vi"("error in (no error)"=w190, "Message Queue"=w191) -> ()  [unwired: 8 in, 2 out]
      }
    }
    frame Error {
    }
  }
  "Need Update" <- w25
  "Feed Module State Cluster out" <- w19
  n109 = local write "Started"(w8) -> ()
  n110 = Release Queue(queue=w6, error in (no error)=w5) -> (error out=→"error out":errorcluster)  [unwired: 1 in, 2 out]
